vi "set_config_cluster.vi"(8 "error in (no error)":errorcluster, 10 "config cluster variant":variant, 11 "TrajectoryAK101022Resonance in":refnum<class "TrajectoryAK101022Resonance.lvclass">) -> (0 "error out":errorcluster, 3 "TrajectoryAK101022Resonance out":refnum<class "TrajectoryAK101022Resonance.lvclass">)   [LabVIEW 2010, in "TrajectoryAK101022Resonance.lvclass"]
uses:
  TrajectoryAK101022Resonance.lvclass
  TrajectoryAK101022Resonance.lvclass/TrajectoryAK101022Resonance.ctl
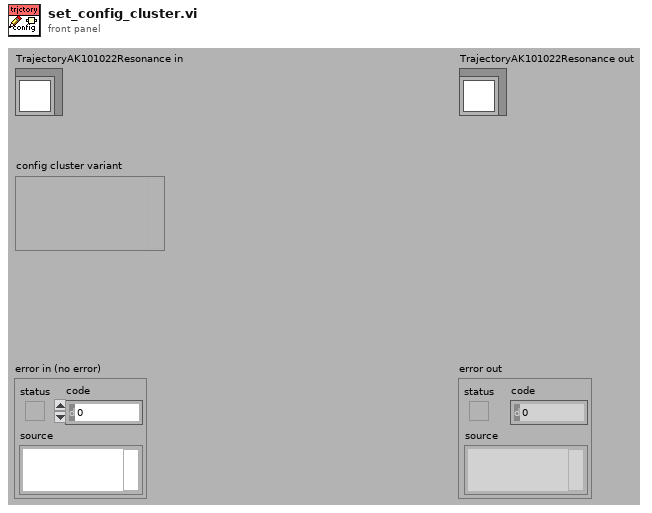
[diagram p1: front panel]
types:
  T1 = typedef "TrajectoryAK101022Resonance.lvclass/config_data_cluster.ctl" = cluster{"resonance frequency":dbl[unit], "no. of y-brake lines before flyback":i32, "no. of y-flyback lines":i32, "no. of y-brake lines after flyback":i32, "maximum x scanner value":dbl, "maximum y scanner value":dbl, "fly-forward offset default":dbl, "fly-back offset default":dbl, "scan segment default":dbl, "FOVx":dbl[unit], "FOVy":dbl[unit], "objective magnification":dbl, "component specification":T2, "number of y-fly-back steps":u16, "ETL current to Hifo-Box conversion":dbl[unit], "ETL current offset":dbl[unit]}
  T2 = typedef "plugin_specification.ctl" = cluster{"class path":string, "configuration":string, "label":string, "settings name":string}
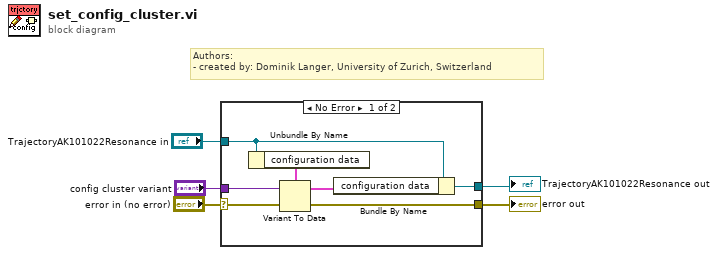
[diagram p0: block diagram]
diagram:
  # "Authors: \n- created by: Dominik Langer, University of Zurich, Switzerland"
  n1 = case shown="No Error" "error in (no error)" {
    selector: "error in (no error)" -> [w6 w13]
    tunnel: "config cluster variant" -> [w12 _]
    tunnel: "TrajectoryAK101022Resonance in" -> [w10 w14]
    tunnel: [w8 w13] -> w3
    tunnel: [w7 w14] -> w2
    frame No Error {
      n2 = Unbundle By Name(w10) -> ("configuration data"=w11:T1)
      n3 = Variant To Data(error in=w6, Variant=w12, type=w11) -> (error out=w8:errorcluster, data=w9:T1)
      n4 = Bundle By Name(cluster=w10, "configuration data"=w9) -> (w7:refnum<class "TrajectoryAK101022Resonance.lvclass">)
    }
    frame Error {
    }
  }
  "error out" <- w3
  "TrajectoryAK101022Resonance out" <- w2
